vi "Simple Example.vi"() -> ()   [LabVIEW 2019]
uses:
  Log/Log.lvclass
  Log Sinks/Sink-Console/Sink-Console.lvclass
  Log Sinks/Sink-Console/Construct - Input.vi
  Log/Event Level.ctl
  TSC Event Logger.lvlib
  Log Sinks/Text File/Text File.lvclass
  C:/Development/Reuse-libraries/Event Logger/Log Sinks/Log Sinks.lvclass
  Log Sinks/Text File/Construct - File.vi
  Layouts/JSONLayout/JSONLayout.lvclass
  cd0cdadd-5bba-4876-b4a7-6d6dc25bebc9.vi
  0255d82c-ae35-4f1c-bf70-cf29c14a7855.vi
  d915b4c3-683c-4e5b-a72c-46a47fdfc3fe.vi
  C:/Development/Reuse-libraries/Event Logger/Layouts/Layout.lvclass
panel:
  in  "Record Event with multiple arg":bool
  in  "Record Event with arg":bool
  in  "Argument List":string[](array[string])
  in  "Single Argument":string
  in  "Add JSON Console":bool
  out "Second Console":string
  out "String":string
  in  "Level":T1=enum."INFO"
  in  "Record Event":bool
  in  "Event Data":string="test"
  out "Error Out":errorcluster
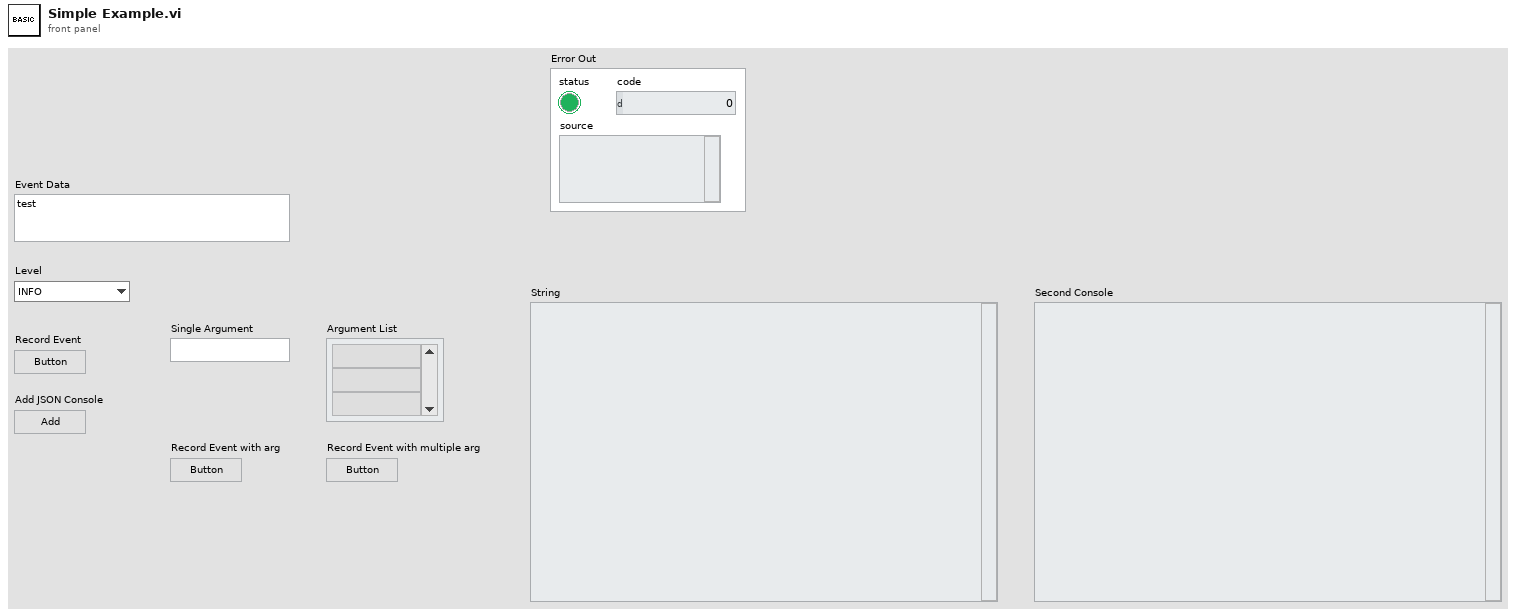
[diagram p1: front panel]
types:
  T1 = typedef "TSC Event Logger.lvlib/Event Level.ctl" = enum16{"OFF", "TRACE", "DEBUG", "INFO", "WARN", "ERROR", "FATAL"}
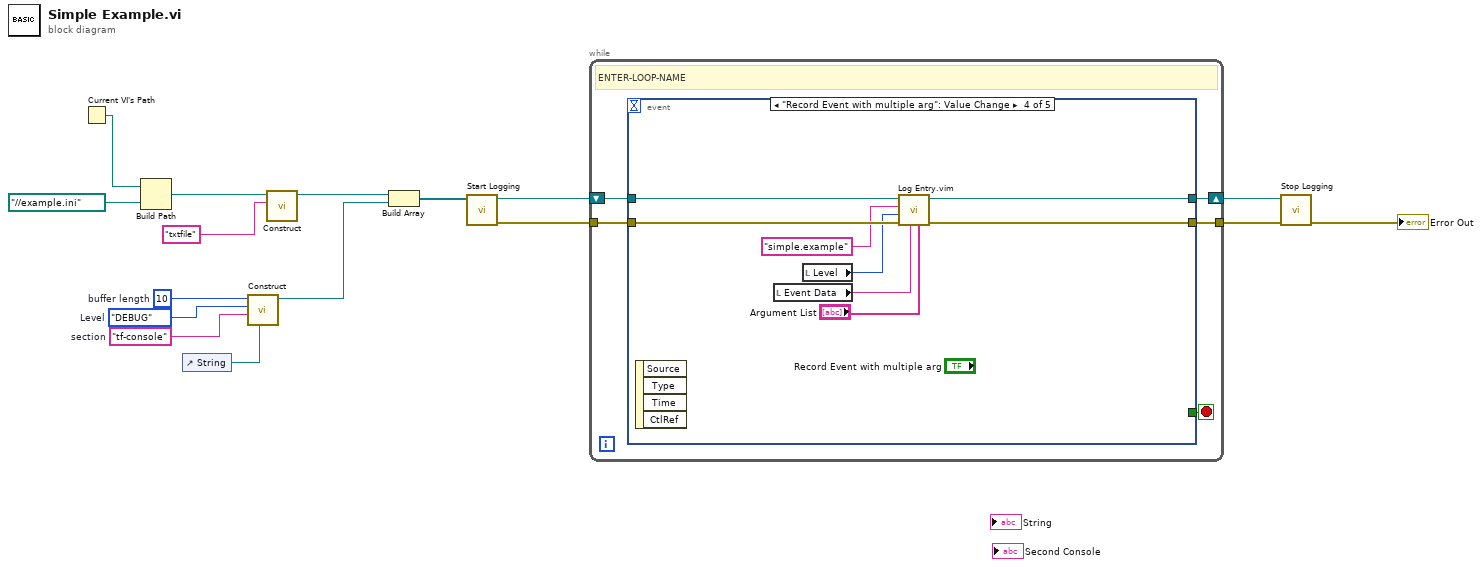
[diagram p0: block diagram]
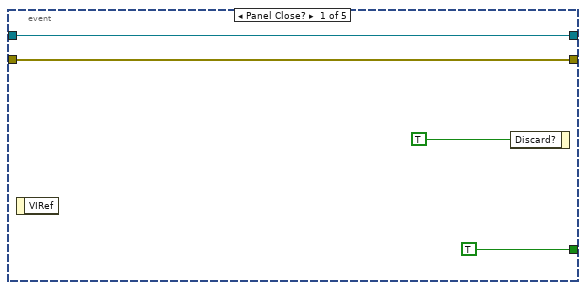
[diagram p2: hidden frame]
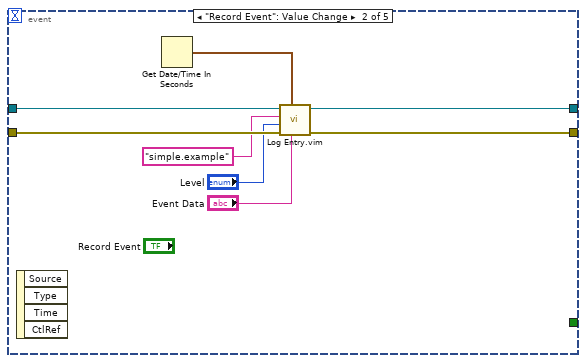
[diagram p3: hidden frame]
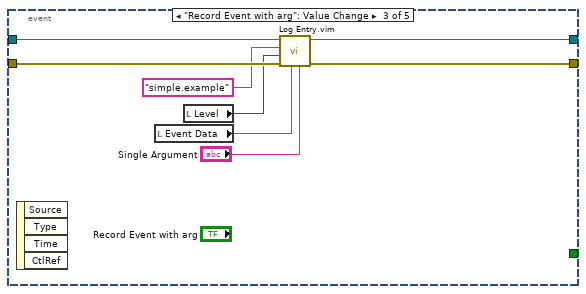
[diagram p4: hidden frame]
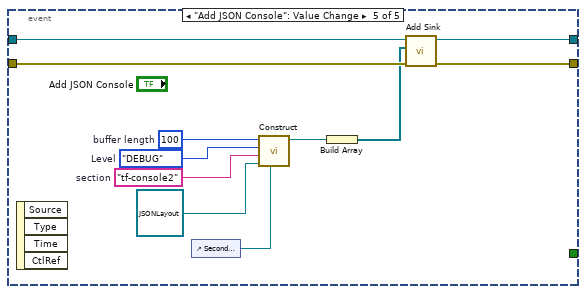
[diagram p5: hidden frame]
diagram:
  w1 = 10  # buffer length
  w2 = Event_Level."DEBUG"  # Level
  w3 = "tf-console"  # section
  n1 = Current VI's Path() -> (path=w8:path)
  n2 = Build Path(base path=w8, name or relative path=path "../../example.ini") -> (appended path=w6:path)
  n3 = control-ref of="String"() -> (w4:refnum<vi>)
  n4 = call-poly "Construct.vi"("Console Ref"=w4, "Name"=w3, "Level"=w2, "buffer length"=w1) -> ("Sink-Console"=w5:refnum<class "Sink-Console.lvclass">)  [unwired: 6 in, 1 out]
  n5 = call-poly "Construct.vi"("section"="txtfile", "config file"=w6) -> ("Text File"=w10:refnum<class "Text File.lvclass">)  [unwired: 8 in, 1 out]
  n6 = Build Array(w10, w5) -> (w9:refnum<class "Log Sinks.lvclass">[])
  n7 = call "Start Logging.vi"("Sinks"=w9) -> ("Error Out"=w15:errorcluster, "Logger"=w12:refnum<class "Log.lvclass">)  [unwired: 9 in]
  n8 = while {
    tunnel: w15 -> [w20]
    shift-right: [w18] -> w14
    shift-left: w12 -> [w19]
    tunnel: [w17] -> w13
    stop <- w21 stop-if-true
    # "ENTER-LOOP-NAME"
    n9 = event shown="[3] \"Record Event with multiple arg\": Value Change" {
      selector: _ -> [_ _ _ _ _]
      dyn-events: _ -> [_ _ _ _ _]
      timeout: _ -> [_ _ _ _ _]
      tunnel: [TRUE _ _ _ _] -> w21
      tunnel: w20 -> [w22 w31 w39 w47 w60]
      tunnel: w19 -> [w23 w33 w41 w49 w58]
      tunnel: [w23 w32 w40 w48 w57] -> w18
      tunnel: [w22 w30 w38 w46 w59] -> w17
      event Panel Close? {
        n10 = event-data() -> ()  [unwired: 1 in, 1 out]
        n11 = event-data("Discard?"=TRUE) -> ()  [unwired: 1 in, 1 out]
      }
      event "Record Event": Value Change {
        n12 = event-data() -> ()  [unwired: 1 in, 4 out]
        n13 = Get Date/Time In Seconds() -> (seconds since 1Jan1904=w28:timestamp)
        n14 = call "Log Entry.vim"("Message"="Event Data", "Time"=w28, "error in (no error)"=w31, "Level"="Level", "Logger"="simple.example", "Log in"=w33) -> ("error out"=w30:errorcluster, "Log out"=w32:refnum<class "Log.lvclass">)  [unwired: 4 in]
      }
      event "Record Event with arg": Value Change {
        n15 = event-data() -> ()  [unwired: 1 in, 4 out]
        n16 = local read "Event Data"() -> (w35:string)
        n17 = local read "Level"() -> (w36:T1)
        n18 = call "Log Entry.vim"("Arguments"="Single Argument", "Message"=w35, "error in (no error)"=w39, "Level"=w36, "Logger"="simple.example", "Log in"=w41) -> ("error out"=w38:errorcluster, "Log out"=w40:refnum<class "Log.lvclass">)  [unwired: 4 in]
      }
      event "Record Event with multiple arg": Value Change {
        n19 = event-data() -> ()  [unwired: 1 in, 4 out]
        n20 = local read "Event Data"() -> (w43:string)
        n21 = local read "Level"() -> (w44:T1)
        n22 = call "Log Entry.vim"("Arguments"="Argument List", "Message"=w43, "error in (no error)"=w47, "Level"=w44, "Logger"="simple.example", "Log in"=w49) -> ("error out"=w46:errorcluster, "Log out"=w48:refnum<class "Log.lvclass">)  [unwired: 4 in]
      }
      event "Add JSON Console": Value Change {
        w56 = 100  # buffer length
        w55 = Event_Level."DEBUG"  # Level
        w54 = "tf-console2"  # section
        n23 = event-data() -> ()  [unwired: 1 in, 4 out]
        n24 = control-ref of="Second Console"() -> (w53:refnum<vi>)
        n25 = call-poly "Construct.vi"("Console Ref"=w53, "Layout Type"=refnum<class "JSONLayout.lvclass"> refnum ("TSC Event Logger.lvlib:JSONLayout.lvclass"), "Name"=w54, "Level"=w55, "buffer length"=w56) -> ("Sink-Console"=w52:refnum<class "Sink-Console.lvclass">)  [unwired: 5 in, 1 out]
        n26 = Build Array(w52) -> (w51:refnum<class "Sink-Console.lvclass">[])
        n27 = call "Add Sink.vi"("Error In"=w60, "Sinks"=w51, "Logger in"=w58) -> ("Error Out"=w59:errorcluster, "Logger"=w57:refnum<class "Log.lvclass">)  [unwired: 7 in]
      }
    }
  }
  n28 = call "Stop Logging.vi"("Error In"=w13, "Logger"=w14) -> ("Error Out"=→"Error Out":errorcluster)  [unwired: 8 in, 1 out]
